vi "Clear Action Core.vi"(8 "error in (no error)":errorcluster, 11 "NI DMM in":refnum<class "NI DMM.lvclass">) -> (0 "error out":errorcluster, 3 "NI DMM out":refnum<class "NI DMM.lvclass">)   [LabVIEW 2020, in "NI DMM.lvlib" / "NI DMM.lvclass"]
uses:
  NI DMM.lvclass
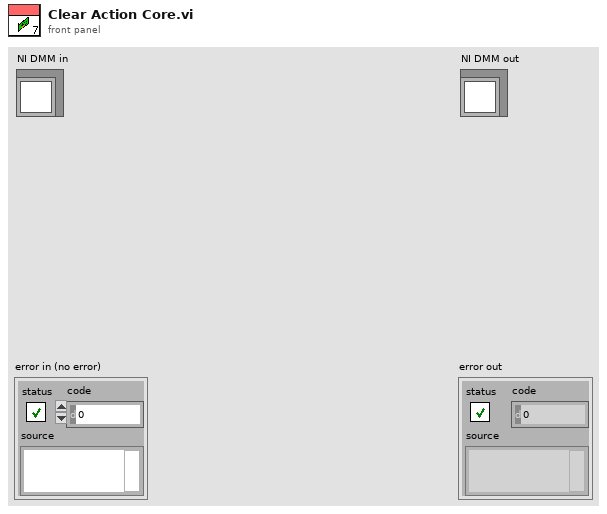
[diagram p1: front panel]
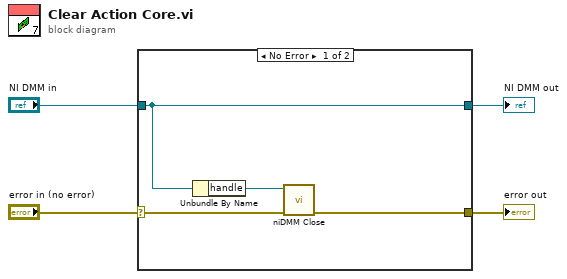
[diagram p0: block diagram]
diagram:
  n1 = case shown="No Error" "error in (no error)" {
    selector: "error in (no error)" -> [w7 w10]
    tunnel: [w5 w10] -> w2
    tunnel: "NI DMM in" -> [w8 w9]
    tunnel: [w8 w9] -> w3
    frame No Error {
      n2 = Unbundle By Name(w8) -> ("handle"=w6:refnum<k15>)
      n3 = call <instrlib>:"niDMM Close.vi"("error in (no error)"=w7, "instrument handle"=w6) -> ("error out"=w5:errorcluster)  [unwired: 9 in]
    }
    frame Error {
    }
  }
  "error out" <- w2
  "NI DMM out" <- w3
